vi "REPORT_select_path_for_pdf_report.vi"(8 "error_in":errorcluster caption="error out", 11 "report_title":string) -> (0 "error_out":errorcluster, 2 "cancelled":bool, 3 "path_to_report":path)   [LabVIEW 2019]
uses:
  _misc/AULocalize/SubVIs/Get Localized Phrase Compact Interface 0D.vi
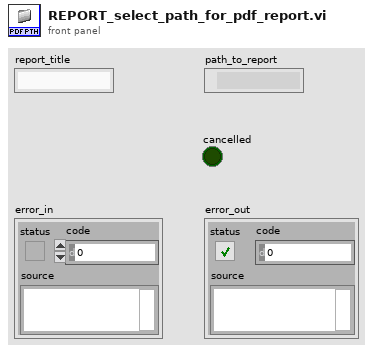
[diagram p1: front panel]
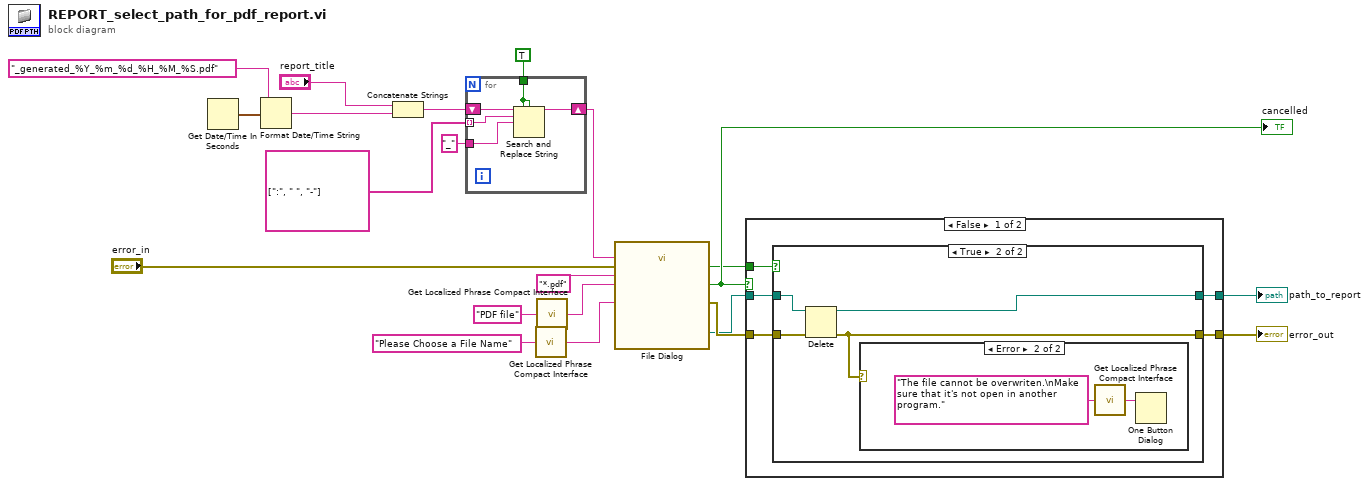
[diagram p0: block diagram]
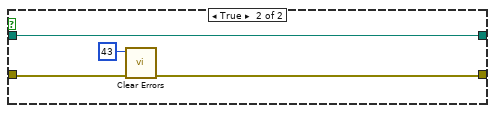
[diagram p4: hidden frame]
diagram:
  n1 = Get Date/Time In Seconds() -> (seconds since 1Jan1904=w13:timestamp)
  n2 = Format Date/Time String(time format string (%c)="_generated_%Y_%m_%d_%H_%M_%S.pdf", seconds (now)=w13) -> (date/time string=w12:string)  [unwired: 1 in]
  n3 = Concatenate Strings("report_title", w12) -> (w7:string)
  n4 = for {
    tunnel: TRUE ("replace all? (F)") -> [w25]
    shift-right: [w24] -> w5
    shift-left: w7 -> [w26]
    tunnel: string[] [":", " ", "-"] -> [w23] mode=indexing
    tunnel: "_" -> [w22]
    n5 = Search and Replace String(replace all?=w25, case sensitive?=w25, input string=w26, search string=w23, replace string=w22) -> (result string=w24:string)  [unwired: 3 in, 3 out]
  }
  n6 = call-poly "Get Localized Phrase Compact Interface.vi"("Key"="Please Choose a File Name" ("prompt")) -> ("Translated Phrase"=w2:string)
  n7 = call-poly "Get Localized Phrase Compact Interface.vi"("Key"="PDF file" ("pattern label")) -> ("Translated Phrase"=w1:string)
  n8 = call "File Dialog"("prompt"=w2, "default name"=w5, "error in"="error_in", "pattern (all files)"="*.pdf", "pattern label"=w1) -> ("selected path"=w15:path, "exists"=w17:bool, "cancelled"=w18:bool, "error out"=w16:errorcluster)  [unwired: 2 in, 5 out]
  "cancelled" <- w18
  n9 = case shown="False" w18 {
    tunnel: w17 -> [w31 _]
    tunnel: w16 -> [w30 w41]
    tunnel: w15 -> [w29 w43]
    tunnel: [w28 w40] -> w9
    tunnel: [w27 w43] -> w10
    frame False {
      n10 = case shown="True" w31 {
        tunnel: w30 -> [w32 w37]
        tunnel: w29 -> [w33 w36]
        tunnel: [w32 w34] -> w28
        tunnel: [w33 w35] -> w27
        frame False {
        }
        frame True {
          n11 = Delete(path (use dialog)=w36, error in=w37) -> (deleted path=w35:path, error out=w34:errorcluster)  [unwired: 4 out]
          n12 = case shown="Error" w34 {
            frame No Error {
            }
            frame Error {
              n13 = call-poly "Get Localized Phrase Compact Interface.vi"("Key"="The file cannot be overwriten.\nMake sure that it's not open in another program." ("prompt")) -> ("Translated Phrase"=w38:string)
              n14 = One Button Dialog(message=w38) -> ()  [unwired: 2 out]
            }
          }
        }
      }
    }
    frame True {
      n15 = call <vilib>:"Clear Errors.vi"("error in (no error)"=w41, "specific error code to clear (0: all)"=43) -> ("error out"=w40:errorcluster)  [unwired: 4 in, 1 out]
    }
  }
  "path_to_report" <- w10
  "error_out" <- w9
